vi "select_temperature_value.vi"() -> ()   [LabVIEW 2019]
uses:
  global_temperature_cluster.ctl
panel:
  in  "Numeric":dbl
  in  "Temperature-Cluster":T1
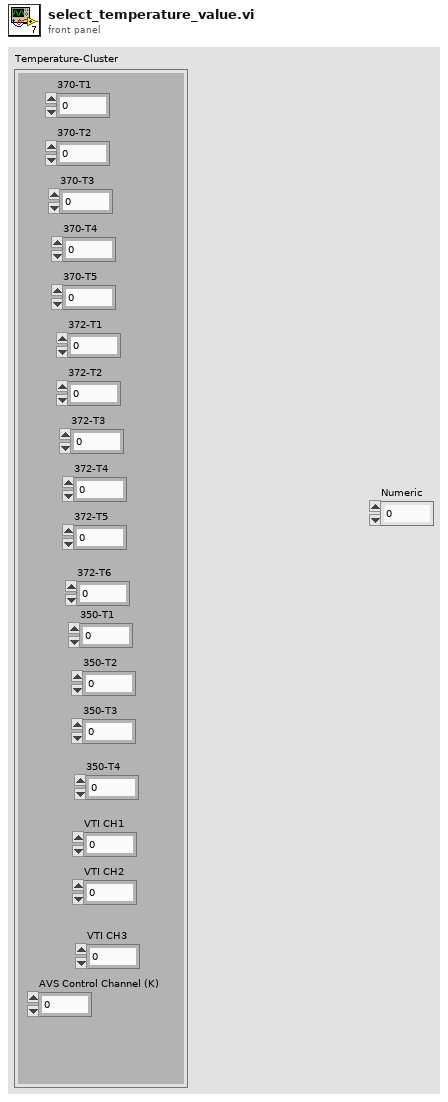
[diagram p1: front panel]
types:
  T1 = typedef "global_temperature_cluster.ctl" = cluster{"370-T1":dbl, "370-T2":dbl, "370-T3":dbl, "370-T4":dbl, "370-T5":dbl, "372-T1":dbl, "372-T2":dbl, "372-T3":dbl, "372-T4":dbl, "372-T5":dbl, "372-T6":dbl, "350-T1":dbl, "350-T2":dbl, "350-T3":dbl, "350-T4":dbl, "VTI CH1":dbl, "VTI CH2":dbl, "VTI CH3":dbl, "AVS Control Channel (K)":dbl}
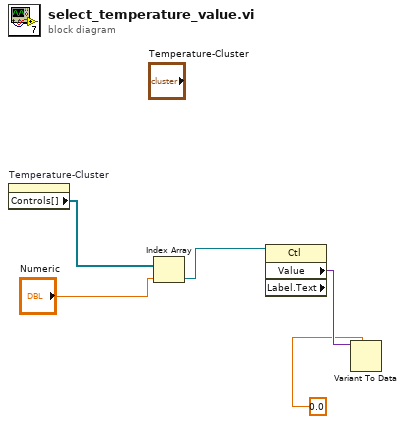
[diagram p0: block diagram]
diagram:
  n1 = property on="Temperature-Cluster" class="Clust (strict)"() -> ("Controls[]"=w5:refnum<vi>[])  [unwired: 2 in, 2 out]
  n2 = Index Array(array=w5, index="Numeric") -> (element=w3:refnum<vi>)
  n3 = property class="Ctl" props=["Value", "Label", "Text"](reference=w3) -> ("Value"=w2:variant)  [unwired: 1 in, 3 out]
  n4 = Variant To Data(type=0.0, Variant=w2) -> ()  [unwired: 1 in, 2 out]
